vi "Get Measurement Details.vi"(8 "error in":errorcluster) -> (0 "error out":errorcluster, 3 "measurement_details":T1)   [LabVIEW 2020, in "LineRegulation.lvlib"]
uses:
  LineRegulation.lvlib
  Service/RPC Messages/Measurement_v1_MeasurementDetails/Measurement_v1_MeasurementDetails_Data.ctl
  Service/MeasurementService_Template.lvclass
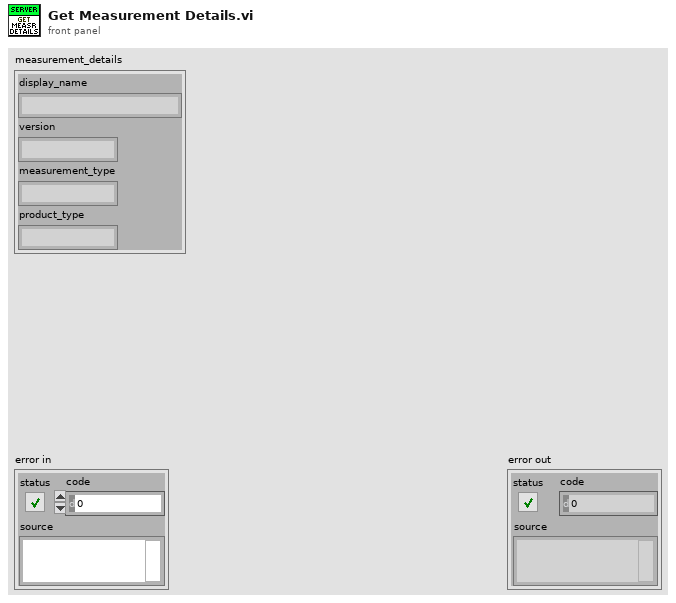
[diagram p1: front panel]
types:
  T1 = typedef "LineRegulation.lvlib/MeasurementService_Template.lvclass/Measurement_v1_MeasurementDetails_Data.ctl" = cluster{"display_name":string, "version":string, "measurement_type":string, "product_type":string}
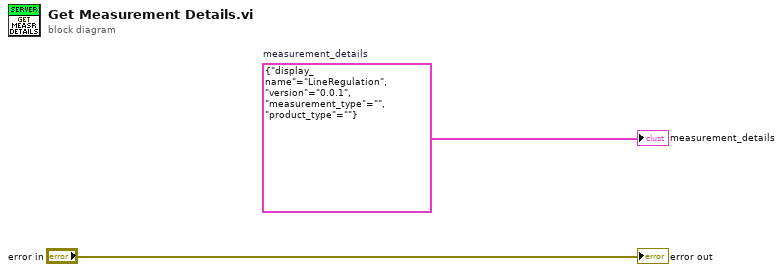
[diagram p0: block diagram]
diagram:
  w1 = T1 {"display_name"="LineRegulation", "version"="0.0.1", "measurement_type"="", "product_type"=""}  # measurement_details
  "error out" <- "error in"
  "measurement_details" <- w1
